vi "AOL Z-stack duration.vi"(10 "Function":T1) -> (3 "AOL z-stack duration (sec)":dbl)   [LabVIEW 2017]
uses:
  Typedefs/Read Write Enum.ctl
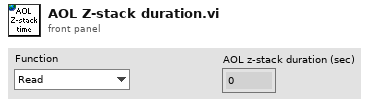
[diagram p1: front panel]
types:
  T1 = typedef "Read Write Enum.ctl" = enum16{"Read", "Write"}
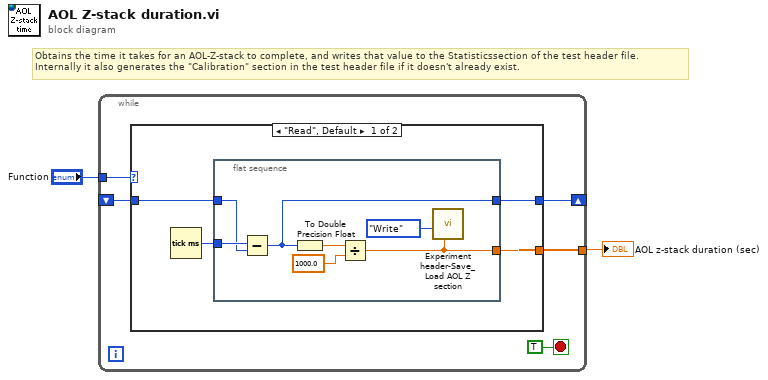
[diagram p0: block diagram]
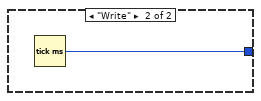
[diagram p2: hidden frame]
diagram:
  # "Obtains the time it takes for an AOL-Z-stack to complete, and writes that value to the Statisticssection of the test header file.\nInternally it also generates the \"Calibration\" section in the test header file if it doesn't already exist."
  n1 = while {
    tunnel: "Function" -> [w7]
    shift-right: [w5] -> _
    shift-left: _ -> [w4]
    tunnel: [w3] -> w1
    stop <- TRUE stop-if-true
    n2 = case shown="\"Read\", Default" w7 {
      tunnel: [w9 w19] -> w5
      tunnel: w4 -> [w10 _]
      tunnel: [w8 _] -> w3
      frame "Read", Default {
        n3 = Tick Count (ms)() -> (millisecond timer value=w11:u32)
        n4 = flat-sequence {
          tunnel: w11 -> [w18]
          tunnel: w10 -> [w17]
          tunnel: [w16] -> w9
          tunnel: [w12] -> w8
          frame #0 {
            n5 = Subtract(x=w18, y=w17) -> (x-y=w16:u32)
            n6 = To Double Precision Float(number=w16) -> (double precision float=w14:dbl)
            n7 = Divide(x=w14, y=1000.0) -> (x/y=w12:dbl)
            n8 = call "Experiment header-Save_Load AOL Z section.vi"("AOL z-stack duration (sec)"=w12, "Function"=enum16{"Write", "Read"}."Write") -> ()  [unwired: 9 in, 1 out]
          }
        }
      }
      frame "Write" {
        n9 = Tick Count (ms)() -> (millisecond timer value=w19:u32)
      }
    }
  }
  "AOL z-stack duration (sec)" <- w1
